vi "Motor.vi"(7 "Boolean":bool=TRUE, 10 "vel":dbl format="%#_13g", 11 "Motor":cluster{"2":bool, "3":bool, "0":bool, "1":bool}={"2"=TRUE, "3"=FALSE, "0"=FALSE, "1"=FALSE}) -> (2 "appended array":string[](array[string]))   [LabVIEW 2018]
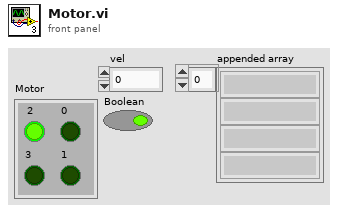
[diagram p1: front panel]
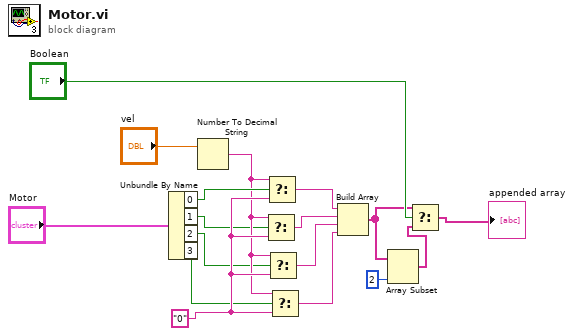
[diagram p0: block diagram]
diagram:
  w15 = "0"
  n1 = Unbundle By Name("Motor") -> ("0"=w16:bool, "1"=w8:bool, "2"=w7:bool, "3"=w6:bool)
  n2 = Number To Decimal String(number="vel") -> (decimal integer string=w14:string)  [unwired: 1 in]
  n3 = Select(t=w14, s=w8, f=w15) -> (s? t:f=w11:string)
  n4 = Select(t=w14, s=w16, f=w15) -> (s? t:f=w12:string)
  n5 = Select(t=w14, s=w7, f=w15) -> (s? t:f=w10:string)
  n6 = Select(t=w14, s=w6, f=w15) -> (s? t:f=w9:string)
  n7 = Build Array(w12, w11, w10, w9) -> (w3:string[])
  n8 = Array Subset(array=w3, length=2) -> (w1:string[])  [unwired: 1 in]
  n9 = Select(t=w3, s="Boolean", f=w1) -> (s? t:f=→"appended array":string[])
